vi "Get Device_Com_Port.vi"(8 "error in (no error)":errorcluster caption="entrée d'erreur (pas d'erreur)", 11 "Class DIO en entrée":refnum<class "Class Instrument Ana.lvclass">) -> (0 "error out":errorcluster caption="sortie d'erreur", 2 "Device_Com_Port":string, 3 "Class DIO en Sortie":refnum<class "Class Instrument Ana.lvclass">)   [LabVIEW 2020, in "Library Instrument & Equipement.lvlib" / "Library Instruments.lvlib" / "Class Instrument Ana.lvclass"]
uses:
  Class Instrument Ana.lvclass
  Class Instrument Ana.lvclass/Class Instrument Ana.ctl
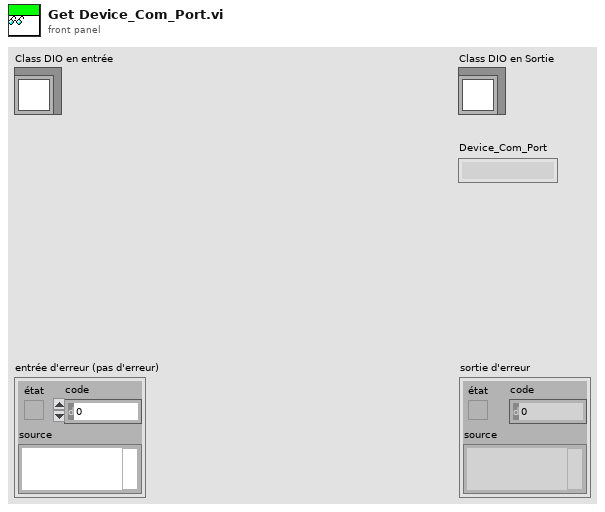
[diagram p1: front panel]
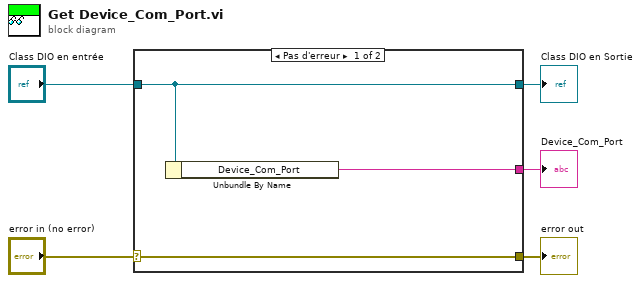
[diagram p0: block diagram]
diagram:
  n1 = case shown="Pas d'erreur" "error in (no error)" {
    selector: "error in (no error)" -> [w8 w9]
    tunnel: [w8 w9] -> w4
    tunnel: [w7 w10] -> w2
    tunnel: "Class DIO en entrée" -> [w7 w10]
    tunnel: [w6 _] -> w1
    frame No Error {
      n2 = Unbundle By Name(w7) -> ("Device_Com_Port"=w6:string)
    }
    frame Error {
    }
  }
  "error out" <- w4
  "Class DIO en Sortie" <- w2
  "Device_Com_Port" <- w1
